vi "Get Replay Data From File.vi"(8 "error in (no error)":errorcluster, 10 "Position reference":T1, 11 "Item Ref in":T2 format="%.0x") -> (0 "error out":errorcluster, 2 "DBL Data":dbl[](array[numeric]), 3 "DAC Data":i16[](array[numeric]))   [LabVIEW 2013, in "Engine Simulation Toolkit System Explorer.lvlib"]
uses:
  Engine Simulation Toolkit System Explorer.lvlib
  <vilib>/NI Veristand/Custom Device API/Custom Device Item Ref.ctl
  Position Reference.ctl
  Data Replay Data Selection Method.ctl
  FPGA Mem Size.ctl
  Shared/Properties.vi
  <vilib>/NI Veristand/Custom Device API/Get Item Property (U16).vi
  <vilib>/NI Veristand/Custom Device API/Get Item Property (Double).vi
  <vilib>/NI Veristand/Custom Device API/Get Item Property (Boolean).vi
  <vilib>/NI Veristand/Custom Device API/Get Item Property (String).vi
  <vilib>/NI Veristand/Custom Device API/Get Item Property (U32).vi
  <vilib>/NI Veristand/Custom Device API/Get Item Property (I32).vi
  <vilib>/NI Veristand/Custom Device API/Get Item Property (Dependent File).vi
  <vilib>/NI Veristand/Custom Device API/Custom Device API.lvlib
  Data File Loader/File Interface.lvlib
  Shared/Engine Simulation Toolkit Shared.lvlib
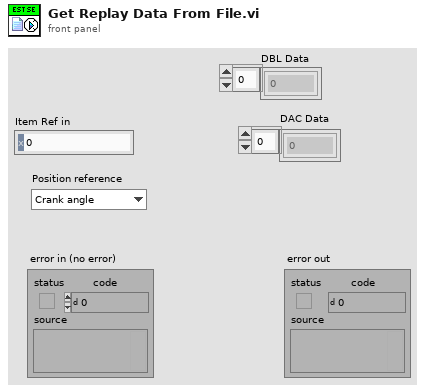
[diagram p1: front panel]
types:
  T1 = typedef "Engine Simulation Toolkit System Explorer.lvlib/Position Reference.ctl" = enum16{"Crank angle", "Cycle angle"}
  T2 = typedef "Custom Device API.lvlib/Custom Device Item Ref.ctl" = u64
  T3 = typedef "Engine Simulation Toolkit System Explorer.lvlib/FPGA Mem Size.ctl" = enum16{"65,536", "32,768", "16,384", "8,192", "4,096", "2,048", "1,024"}
  T4 = typedef "Engine Simulation Toolkit System Explorer.lvlib/Data Replay Data Selection Method.ctl" = enum32{"Manual", "AutoVRCrank"}
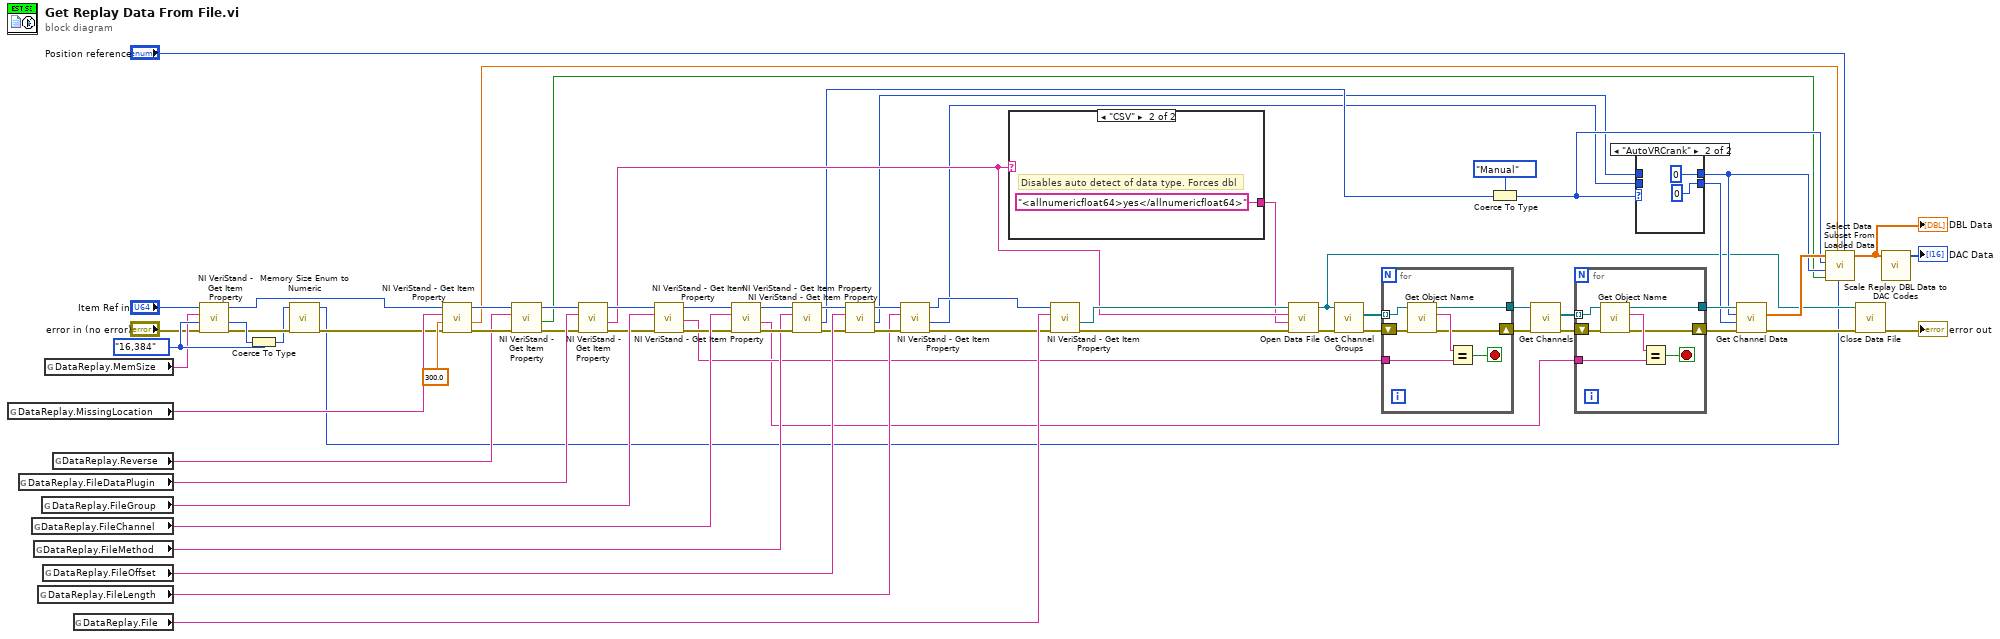
[diagram p0: block diagram]
diagram:
  w10 = FPGA_Mem_Size."16,384" ("FPGA Memory Size")
  n1 = global read "Properties.vi" "DataReplay.MissingLocation"() -> (w66:string)
  n2 = global read "Properties.vi" "DataReplay.FileDataPlugin"() -> (w63:string)
  n3 = global read "Properties.vi" "DataReplay.FileChannel"() -> (w58:string)
  n4 = global read "Properties.vi" "DataReplay.FileMethod"() -> (w54:string)
  n5 = global read "Properties.vi" "DataReplay.FileLength"() -> (w48:string)
  n6 = global read "Properties.vi" "DataReplay.FileGroup"() -> (w61:string)
  n7 = global read "Properties.vi" "DataReplay.FileOffset"() -> (w52:string)
  n8 = global read "Properties.vi" "DataReplay.MemSize"() -> (w6:string)
  n9 = global read "Properties.vi" "DataReplay.Reverse"() -> (w12:string)
  n10 = global read "Properties.vi" "DataReplay.File"() -> (w46:string)
  n11 = call-poly <vilib>:"NI VeriStand - Get Item Property.vi"("error in (no error)"="error in (no error)", "Default Value"=w10, "Property Name"=w6, "Item Ref in"="Item Ref in") -> ("error out"=w8:errorcluster, "Value"=w9:u16, "Item Ref out"=w4:T2)  [unwired: 4 in, 1 out]
  n12 = Coerce To Type(0:w9, 1:w10) -> (2:w7:T3)
  n13 = call "Memory Size Enum to Numeric.vi"("error in (no error)"=w8, "FPGA Memory Size"=w7) -> ("error out"=w5:errorcluster, "Numeric"=w1:i32)  [unwired: 8 in]
  n14 = call-poly <vilib>:"NI VeriStand - Get Item Property.vi"("error in (no error)"=w5, "Default Value"=300.0, "Property Name"=w66, "Item Ref in"=w4) -> ("error out"=w64:errorcluster, "Value"=w26:dbl, "Item Ref out"=w65:T2)  [unwired: 4 in, 1 out]
  n15 = call-poly <vilib>:"NI VeriStand - Get Item Property.vi"("error in (no error)"=w64, "Property Name"=w12, "Item Ref in"=w65) -> ("error out"=w14:errorcluster, "Value"=w11:bool, "Item Ref out"=w13:T2)  [unwired: 5 in, 1 out]
  n16 = call-poly <vilib>:"NI VeriStand - Get Item Property.vi"("error in (no error)"=w14, "Property Name"=w63, "Item Ref in"=w13) -> ("error out"=w60:errorcluster, "Value"=w43:string, "Item Ref out"=w62:T2)  [unwired: 5 in, 1 out]
  n17 = call-poly <vilib>:"NI VeriStand - Get Item Property.vi"("error in (no error)"=w60, "Property Name"=w61, "Item Ref in"=w62) -> ("error out"=w57:errorcluster, "Value"=w38:string, "Item Ref out"=w59:T2)  [unwired: 5 in, 1 out]
  n18 = call-poly <vilib>:"NI VeriStand - Get Item Property.vi"("error in (no error)"=w57, "Property Name"=w58, "Item Ref in"=w59) -> ("error out"=w55:errorcluster, "Value"=w33:string, "Item Ref out"=w56:T2)  [unwired: 5 in, 1 out]
  n19 = call-poly <vilib>:"NI VeriStand - Get Item Property.vi"("error in (no error)"=w55, "Property Name"=w54, "Item Ref in"=w56) -> ("error out"=w51:errorcluster, "Value"=w29:u32, "Item Ref out"=w53:T2)  [unwired: 5 in, 1 out]
  n20 = call-poly <vilib>:"NI VeriStand - Get Item Property.vi"("error in (no error)"=w51, "Property Name"=w52, "Item Ref in"=w53) -> ("error out"=w49:errorcluster, "Value"=w21:i32, "Item Ref out"=w50:T2)  [unwired: 5 in, 1 out]
  n21 = call-poly <vilib>:"NI VeriStand - Get Item Property.vi"("error in (no error)"=w49, "Property Name"=w48, "Item Ref in"=w50) -> ("error out"=w15:errorcluster, "Value"=w22:i32, "Item Ref out"=w47:T2)  [unwired: 5 in, 1 out]
  n22 = case shown="\"CSV\"" w43 {
    tunnel: [_ "<allnumericfloat64>yes</allnumericfloat64>"] -> w42
    frame Default {
    }
    frame "CSV" {
      # "Disables auto detect of data type. Forces dbl"
    }
  }
  n23 = call-poly <vilib>:"NI VeriStand - Get Item Property.vi"("error in (no error)"=w15, "Property Name"=w46, "Item Ref in"=w47) -> ("error out"=w44:errorcluster, "Path"=w45:path)  [unwired: 4 in, 3 out]
  n24 = call "Open Data File.vi"("error in (no error)"=w44, "Additional parameters"=w42, "Data Plugin"=w43, "File Path"=w45) -> ("error out"=w41:errorcluster, "File Ref"=w19:refnum<k20>)  [unwired: 6 in]
  n25 = call "Get Channel Groups.vi"("error in (no error)"=w41, "File Ref in"=w19) -> ("error out"=w40:errorcluster, "Channel Groups"=w39:refnum<k20>[])  [unwired: 7 in, 1 out]
  n26 = for {
    shift-right: [w69] -> w37
    shift-left: w40 -> [w75]
    tunnel: w39 -> [w74] mode=indexing
    tunnel: [w71] -> w36
    tunnel: w38 -> [w70]
    stop <- w72 stop-if-true
    n27 = call "Get Object Name.vi"("error in (no error)"=w75, "Storage Object in"=w74) -> ("error out"=w69:errorcluster, "Name"=w73:string, "Storage Object out"=w71:refnum<k20>)  [unwired: 7 in]
    n28 = Equal?(x=w73, y=w70) -> (x = y?=w72:bool)
  }
  n29 = Coerce To Type(0:w29, 1:Data_Replay_Data_Selection_Method."Manual" ("Data Selection Method")) -> (2:w24:T4)
  n30 = call "Get Channels.vi"("error in (no error)"=w37, "Channel Group in"=w36) -> ("error out"=w35:errorcluster, "Channels"=w34:refnum<k20>[])  [unwired: 7 in, 1 out]
  n31 = for {
    shift-right: [w76] -> w32
    shift-left: w35 -> [w82]
    tunnel: w34 -> [w81] mode=indexing
    tunnel: [w78] -> w31
    tunnel: w33 -> [w77]
    stop <- w79 stop-if-true
    n32 = call "Get Object Name.vi"("error in (no error)"=w82, "Storage Object in"=w81) -> ("error out"=w76:errorcluster, "Name"=w80:string, "Storage Object out"=w78:refnum<k20>)  [unwired: 7 in]
    n33 = Equal?(x=w80, y=w77) -> (x = y?=w79:bool)
  }
  n34 = case shown="\"AutoVRCrank\"" w24 {
    tunnel: [w84 0 ("Count (0: Read All)")] -> w30
    tunnel: [w83 0 ("index")] -> w23
    tunnel: w22 -> [w84 _]
    tunnel: w21 -> [w83 _]
    frame "Manual", Default {
    }
    frame "AutoVRCrank" {
    }
  }
  n35 = call "Get Channel Data.vi"("error in"=w32, "Count (0: Read All)"=w30, "index"=w23, "Channel in"=w31) -> ("error out"=w20:errorcluster, "Signal"=w27:dbl[])  [unwired: 5 in, 1 out]
  n36 = call "Select Data Subset From Loaded Data.vi"("Position reference"="Position reference", "Memory Size as number"=w1, "MissingTeeth"=w26, "ReverseData"=w11, "Offset"=w23, "Data Selection Method"=w24, "Signal"=w27) -> ("Resampled Data"=w18:dbl[])  [unwired: 2 in, 2 out]
  "DBL Data" <- w18
  n37 = call "Close Data File.vi"("error in (no error)"=w20, "File Ref"=w19) -> ("error out"=→"error out":errorcluster)  [unwired: 9 in]
  n38 = call "Scale Replay DBL Data to DAC Codes.vi"("replay data"=w18) -> ("DAC data"=→"DAC Data":i16[])  [unwired: 10 in]
